vi "design01.vi"() -> ()   [LabVIEW 2015]
panel:
  out "Slide":u8(slide) scale=0.0..100.0
  out "x+y":u16
  out "x-y":u8
  in  "Input 2":u8
  in  "Input 1":u8
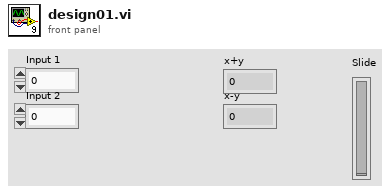
[diagram p1: front panel]
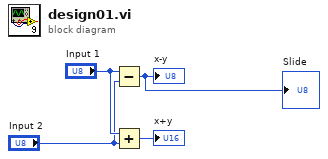
[diagram p0: block diagram]
diagram:
  n1 = Subtract(x="Input 1", y="Input 2") -> (x-y=→"x-y" →"Slide":u8)
  n2 = Add(x="Input 1", y="Input 2") -> (x+y=→"x+y":u8)
